vi "FTP file save.vi"() -> ()   [LabVIEW 2018]
uses:
  <vilib>/FTP/NI_FTP.lvlib
panel:
  in  "host":string="192.168.18.74"
  in  "remote path":string="C:\\Users\\bryan.lee\\Desktop\\"
  in  "OK Button":bool
  in  "stop":bool
  out "data":string
  out "error out":errorcluster
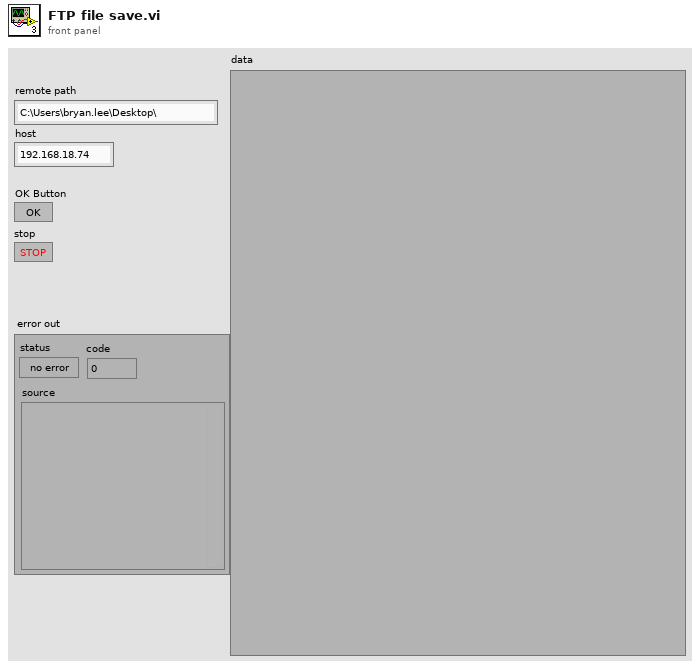
[diagram p1: front panel]
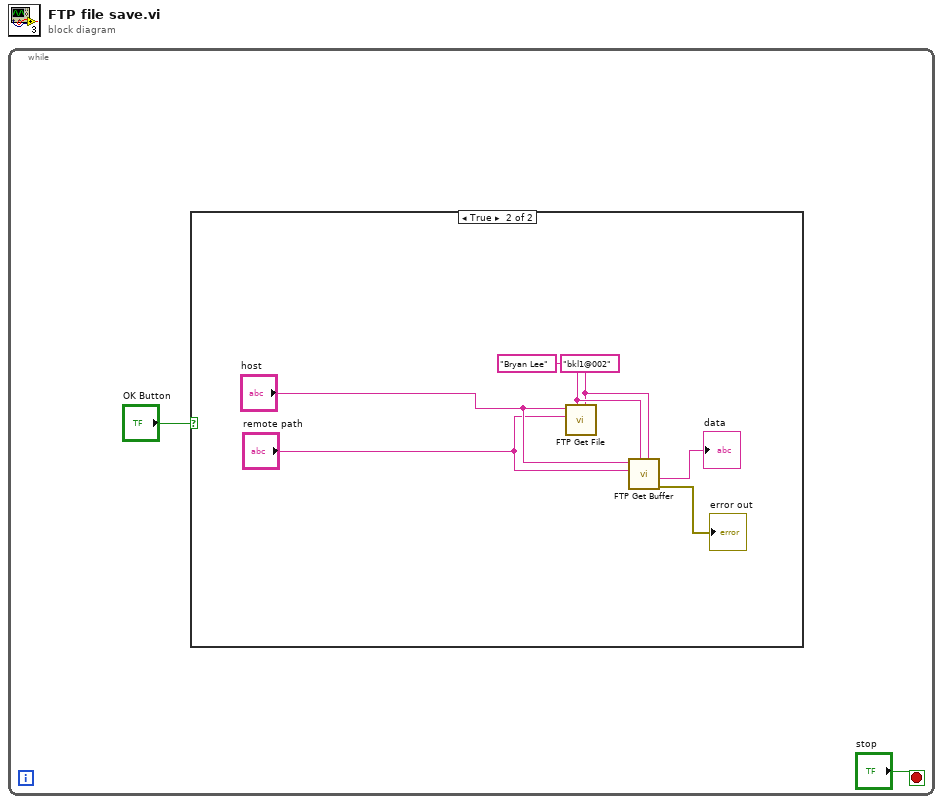
[diagram p0: block diagram]
diagram:
  n1 = while {
    stop <- "stop" stop-if-true
    n2 = case shown="True" "OK Button" {
      frame False {
      }
      frame True {
        w5 = "bkl1@002" ("password")
        w6 = "Bryan Lee" ("user")
        n3 = call <vilib>:"FTP Get File.vi"("password"=w5, "user"=w6, "remote path"="remote path", "host"="host") -> ()  [unwired: 6 in, 2 out]
        n4 = call <vilib>:"FTP Get Buffer.vi"("password"=w5, "user"=w6, "remote path"="remote path", "host"="host") -> ("error out"=→"error out":errorcluster, "data"=→"data":string)  [unwired: 5 in, 1 out]
      }
    }
  }
